vi "AvrgDecimate.vi"(6 "Decimate by":i32, 7 "Average?":bool=TRUE, 11 "waveform":waveform(sgl)={"t0"=timestamp(0 s since 1904-01-01), "dt"=0.0, "Y"=[]}) -> (3 "output waveform":waveform(sgl))   [LabVIEW 2019]
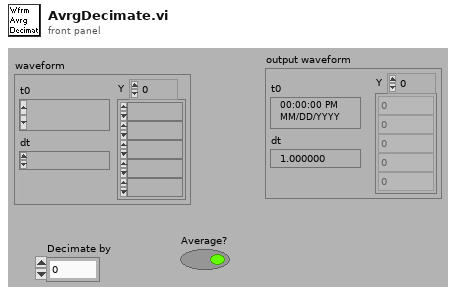
[diagram p1: front panel]
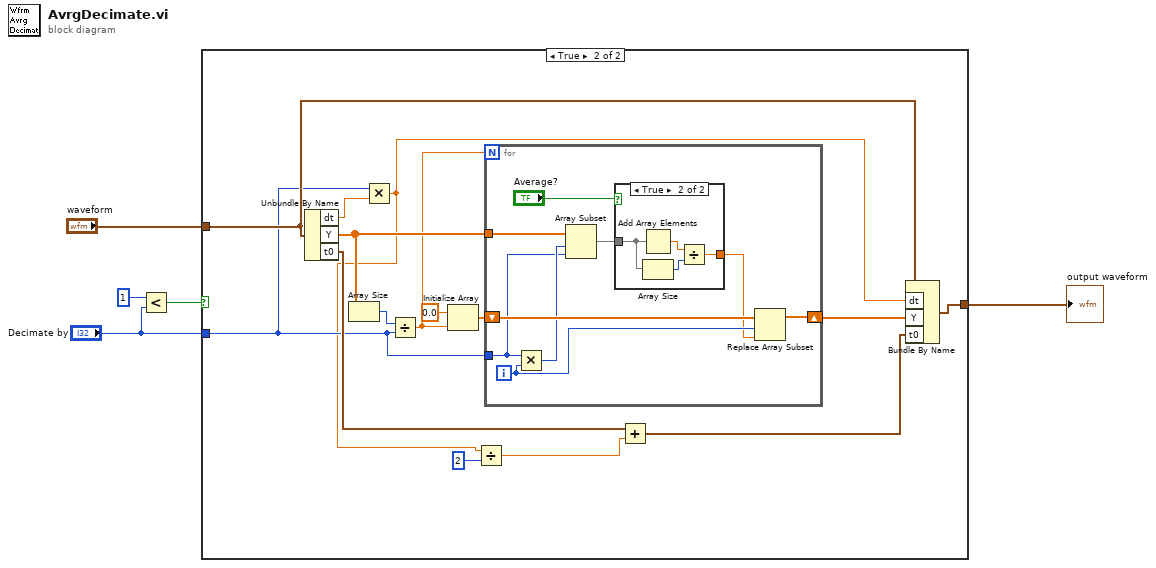
[diagram p0: block diagram]
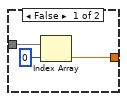
[diagram p3: hidden frame]
diagram:
  n1 = Less?(x=1, y="Decimate by") -> (x < y?=w3:bool)
  n2 = case shown="True" w3 {
    tunnel: "waveform" -> [w6 w16]
    tunnel: "Decimate by" -> [_ w10]
    tunnel: [w6 w13] -> w4
    frame False {
    }
    frame True {
      n3 = Unbundle By Name(w16) -> ("dt"=w15:dbl, "Y"=w21:sgl[], "t0"=w12:timestamp)
      n4 = Array Size(array=w21) -> (size(s)=w20:i32)
      n5 = Multiply(x=w10, y=w15) -> (x*y=w8:dbl)
      n6 = Divide(x=w20, y=w10) -> (x/y=w19:dbl)
      n7 = Initialize Array(sgl 0.0, w19) -> (w17:sgl[])
      n8 = Divide(x=w8, y=2) -> (x/y=w7:dbl)
      n9 = for {
        N: w19 -> [_]
        tunnel: w21 -> [w30]
        shift-right: [w28] -> w14
        shift-left: w17 -> [w29]
        tunnel: w10 -> [w25]
        i -> [w27]
        n10 = Multiply(x=w25, y=w27) -> (x*y=w26:i32)
        n11 = Array Subset(array=w30, index=w26, length=w25) -> (w23:sgl[])
        n12 = case shown="True" "Average?" {
          tunnel: w23 -> [w33 w37]
          tunnel: [w32 w34] -> w22
          frame False {
            n13 = Index Array(array=w33, index=0) -> (element=w32:sgl)
          }
          frame True {
            n14 = Add Array Elements(numeric array=w37) -> (sum=w36:sgl)
            n15 = Array Size(array=w37) -> (size(s)=w35:i32)
            n16 = Divide(x=w36, y=w35) -> (x/y=w34:sgl)
          }
        }
        n17 = Replace Array Subset(array=w29, new element=w22, index=w27) -> (w28:sgl[])
      }
      n18 = Add(x=w12, y=w7) -> (x+y=w11:timestamp)
      n19 = Bundle By Name(cluster=w16, "dt"=w8, "Y"=w14, "t0"=w11) -> (w13:waveform(sgl))
    }
  }
  "output waveform" <- w4
